vi "1762AdiabaticPassageSequenceALLYB.vi"(0 "Interval":dbl=0.02, 1 "Pump Expose Time (us)":dbl=3.0, 5 "Real Cutoff":i32=15, 7 "runs":dbl, 9 "1762 Freq (MHz)":dbl=98.1, 11 "AP Sweep Width (MHz)":dbl=0.8, 12 "Sweep Duration (us)":dbl=500.0, 13 "Power (-12 Max)":dbl=-12.0) -> (4 "Shelved Fraction":dbl=60.0, 6 "Histogram":waveform(i32)(graph)={"t0"=timestamp(22.5 s since 1904-01-01), "dt"=1.0, "Y"=[1, 1, 1, 1, 0, 6, 2, 2, 3, 4, 7, 6, 5, 10, 5, 12, 9, 9, 11, 8, 6, 6, 14, 4, 7, 2, 1, 3, 3, 3, 1, 0, 1, 0, 3, 0, 0, 0, 0, 0, 0, 0, 0, 0, 0, 0, 0, 0, 0, 0, 0, 0, 0, 0, 0, 0, 0, 0, 0, 0, 0, 0, 0, 0, 0, 0, 0, 0, 0, 0, 0, 0, 0, 0, 0, 0, 0, 0, 0, 0, 0, 0, 1, 0, 0, 0, 0, 1, 0, 0, 1, 0, 2, 0, 1, 2, 0, 2, 0, 4, 5, 0, 0, 2, 3, 2, 3, 8, 4, 7, 6, 3, 7, 5, 6, 9, 6, 8, 4, 10, 4, 4, 7, 7, 6, 8, 11, 7, 12, 6, 13, 6, 7, 12, 11, 11, 2, 4, 5, 6, 7, 5, 5, 4, 5, 4, 3, 2, 4, 6, 3, 2, 3, 1, 0, 4, 2, 1, 2, 1, 2, 1, 2, 2, 1, 1, 1, 1, 0, 0, 1, 1, 1, 0, 0, 2, 0, 0, 2]})   [LabVIEW 2009]
uses:
  <vilib>/Utility/file.llb/Write To Spreadsheet File (DBL).vi
panel:
  out "deshelve attempts":dbl
  out "+/-":dbl=0.4472135954999579
  in  "Restart":bool
  out "Shelving Events":dbl=4.0
  out "Cut-off":i32=50
  out "Background":waveform(i32)(graph)={"t0"=timestamp(64.5 s since 1904-01-01), "dt"=1.0, "Y"=[1, 2, 1, 4, 2, 4, 2, 1, 3, 6, 4, 5, 6, 6, 5, 4, 6, 9, 5, 6, 10, 7, 5, 5, 9, 10, 2, 7, 8, 2, 6, 2, 10, 6, 3, 4, 2, 5, 2, 1, 2, 1, 1, 2, 2, 0, 0, 1, 1, 2]}
  out "+ / -":dbl=10.808259218610711
  out "Background":dbl=86.175
  out "Run Number":dbl=6.0
  out "Path":path=path "c:/data/01-11-2009_14-34-35_0.1000001762AdiabaticPass.txt"
  out "Counts":i32=27
  out "Green":bool=TRUE
  out "Shelved?":bool=TRUE
  out "Red":bool=TRUE
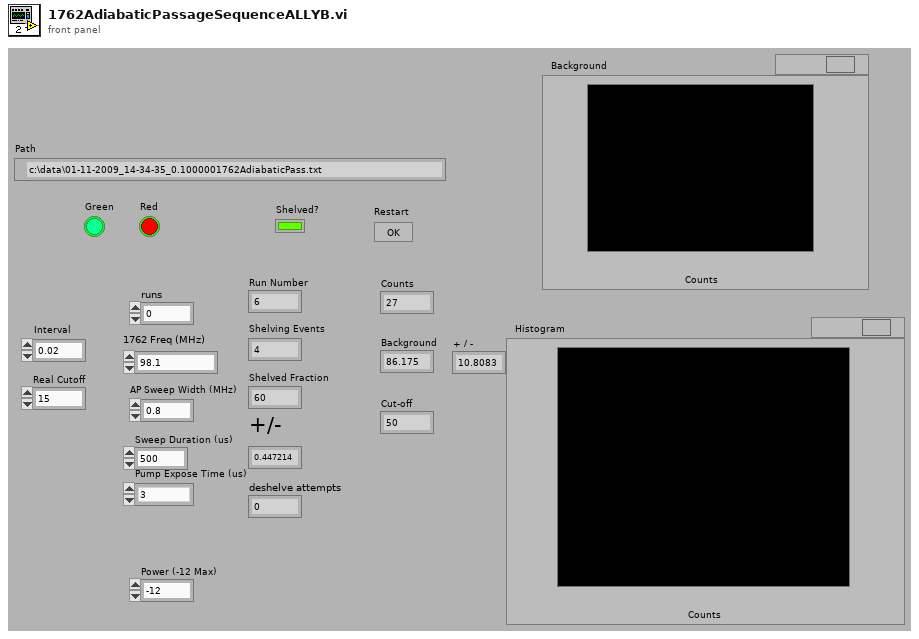
[diagram p1: front panel]
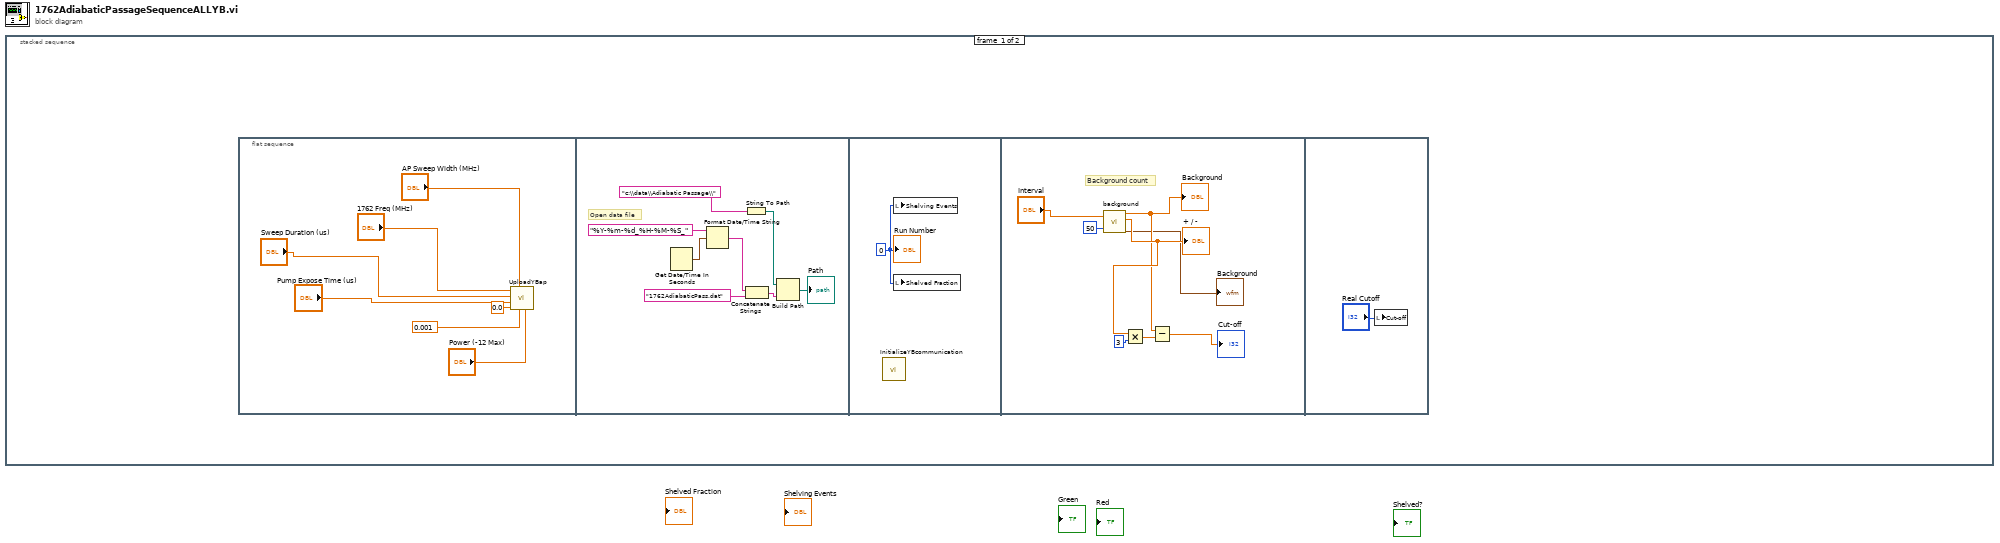
[diagram p0: block diagram]
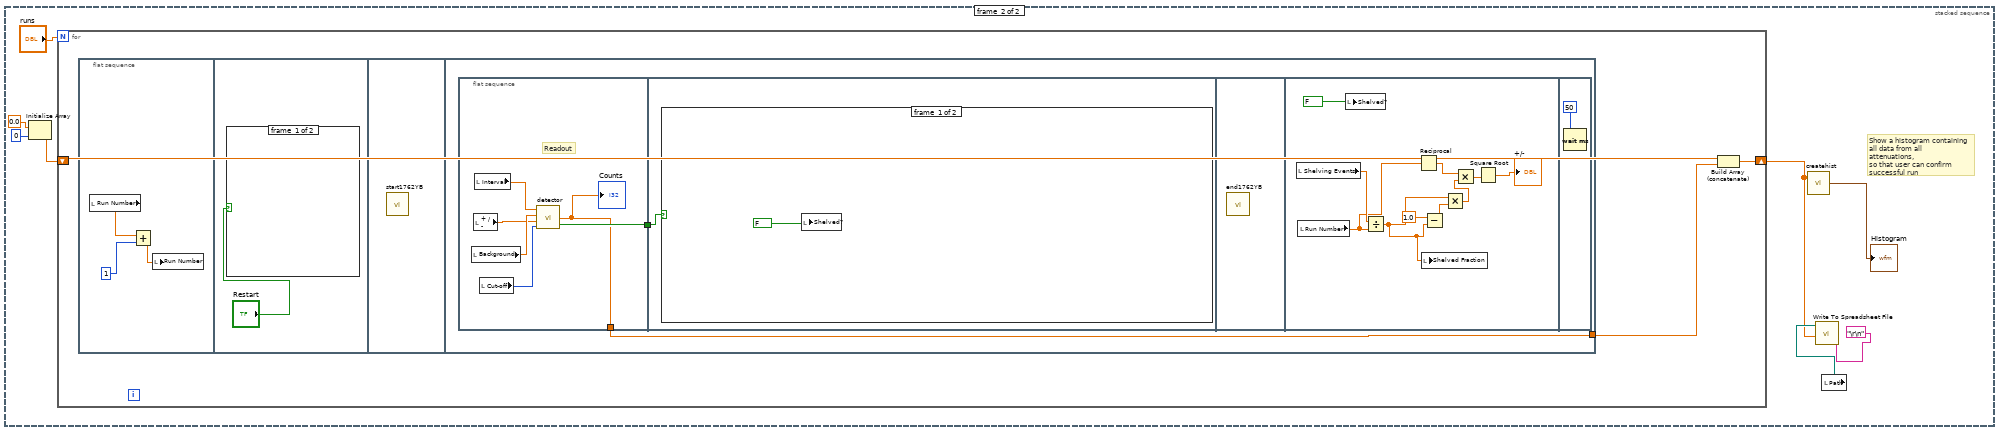
[diagram p2: hidden frame]
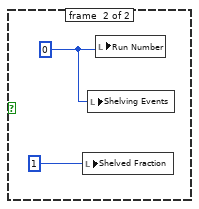
[diagram p3: hidden frame]
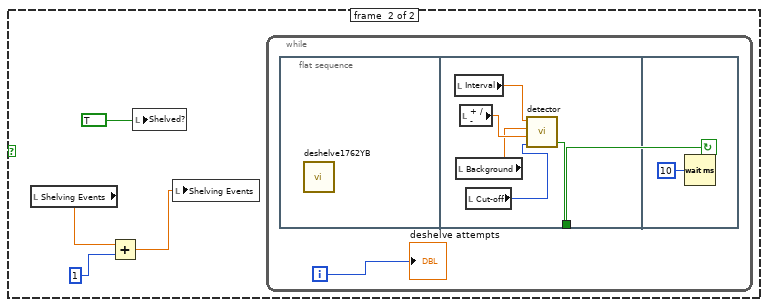
[diagram p4: hidden frame]
diagram:
  n1 = stacked-sequence {
    frame #0 {
      n2 = flat-sequence {
        frame #0 {
          n3 = call "UploadYBap.vi"("Power"="Power (-12 Max)", "AP Freq Step"=0.001, "AP Sweep Width"="AP Sweep Width (MHz)", "1762 RF time"=0.0 ("RF time"), "OP Time"="Pump Expose Time (us)", "1762 Pulse Time"="Sweep Duration (us)", "1762 Frequency"="1762 Freq (MHz)") -> ()  [unwired: 5 in]
        }
        frame #1 {
          # "Open data file"
          n4 = Get Date/Time In Seconds() -> (seconds since 1Jan1904=w13:timestamp)
          n5 = Format Date/Time String(time format string (%c)="%Y-%m-%d_%H-%M-%S_", seconds (now)=w13) -> (date/time string=w15:string)  [unwired: 1 in]
          n6 = String To Path(string="c:\\data\\Adiabatic Passage\\") -> (path=w11:path)
          n7 = Concatenate Strings(w15, "1762AdiabaticPass.dat") -> (w9:string)
          n8 = Build Path(base path=w11, name or relative path=w9) -> (appended path=→"Path":path)
        }
        frame #2 {
          w16 = 0
          n9 = call "InitializeYBcommunication.vi"() -> ()  [unwired: 12 in]
          n10 = local write "Shelving Events"(w16) -> ()
          n11 = local write "Shelved Fraction"(w16) -> ()
          "Run Number" <- w16
        }
        frame #3 {
          # "Background count"
          n12 = call "background.vi"("Interval"="Interval", "Runs"=50) -> ("Mean"=w21:dbl, "Deviation"=w24:dbl, "Histogram"=→"Background":waveform(i32))  [unwired: 1 out]
          "Background" <- w21
          "+ / -" <- w24
          n13 = Multiply(x=w24, y=3) -> (x*y=w22:dbl)
          n14 = Subtract(x=w21, y=w22) -> (x-y=→"Cut-off":dbl)
        }
        frame #4 {
          n15 = local write "Cut-off"("Real Cutoff") -> ()
        }
      }
    }
    frame #1 {
      # "Show a histogram containing\nall data from all attenuations, \nso that user can confirm successful run"
      n16 = Initialize Array(0.0, 0) -> (w29:dbl[])
      n17 = for {
        N: "runs" -> [_]
        shift-right: [w34] -> w27
        shift-left: w29 -> [w35]
        n18 = flat-sequence {
          tunnel: [w43] -> w36
          frame #0 {
            n19 = local read "Run Number"() -> (w37:dbl)
            n20 = Add(x=w37, y=1) -> (x+y=w38:dbl)
            n21 = local write "Run Number"(w38) -> ()
          }
          frame #1 {
            n22 = case shown="True" "Restart" {
              frame #0 {
              }
              frame #1 {
                w42 = 0
                n23 = local write "Shelved Fraction"(1) -> ()
                n24 = local write "Shelving Events"(w42) -> ()
                n25 = local write "Run Number"(w42) -> ()
              }
            }
          }
          frame #2 {
            n26 = call "start1762YB.vi"() -> ()  [unwired: 11 in, 1 out]
          }
          frame #3 {
            n27 = flat-sequence {
              tunnel: [w47] -> w44
              tunnel: [w46] -> w43
              tunnel: w44 -> [w51]
              frame #0 {
                # "Readout"
                n28 = local read "Background"() -> (w50:dbl)
                n29 = local read "+ / -"() -> (w49:dbl)
                n30 = local read "Interval"() -> (w48:dbl)
                n31 = local read "Cut-off"() -> (w45:i32)
                n32 = call "detector.vi"("Cutoff"=w45, "+ / -"=w49, "Background"=w50, "Interval"=w48) -> ("Boolean"=w47:bool, "Counts"=w46:dbl)  [unwired: 1 in]
                "Counts" <- w46
              }
              frame #1 {
                n33 = case shown="True" w51 {
                  frame #0 {
                    n34 = local write "Shelved?"(FALSE) -> ()
                  }
                  frame #1 {
                    n35 = local read "Shelving Events"() -> (w55:dbl)
                    n36 = Add(x=w55, y=1) -> (x+y=w54:dbl)
                    n37 = local write "Shelved?"(TRUE) -> ()
                    n38 = local write "Shelving Events"(w54) -> ()
                    n39 = while {
                      i -> [w57]
                      stop <- w58 continue-if-true
                      n40 = flat-sequence {
                        tunnel: [w63] -> w58
                        frame #0 {
                          n41 = call "deshelve1762YB.vi"() -> ()  [unwired: 11 in, 1 out]
                        }
                        frame #1 {
                          n42 = local read "Interval"() -> (w60:dbl)
                          n43 = local read "Background"() -> (w61:dbl)
                          n44 = local read "+ / -"() -> (w62:dbl)
                          n45 = local read "Cut-off"() -> (w59:i32)
                          n46 = call "detector.vi"("Cutoff"=w59, "+ / -"=w62, "Background"=w61, "Interval"=w60) -> ("Boolean"=w63:bool)  [unwired: 1 in, 1 out]
                        }
                        frame #2 {
                          n47 = Wait (ms)(milliseconds to wait=u32 10) -> ()  [unwired: 1 out]
                        }
                      }
                      "deshelve attempts" <- w57
                    }
                  }
                }
              }
              frame #2 {
                n48 = call "end1762YB.vi"() -> ()  [unwired: 1 in]
              }
              frame #3 {
                n49 = local read "Shelving Events"() -> (w68:dbl)
                n50 = local read "Run Number"() -> (w67:dbl)
                n51 = local write "Shelved?"(FALSE) -> ()
                n52 = Divide(x=w68, y=w67) -> (x/y=w66:dbl)
                n53 = Reciprocal(x=w67) -> (1/x=w73:dbl)
                n54 = local write "Shelved Fraction"(w66) -> ()
                n55 = Subtract(x=1.0, y=w66) -> (x-y=w71:dbl)
                n56 = Multiply(x=w66, y=w71) -> (x*y=w69:dbl)
                n57 = Multiply(x=w73, y=w69) -> (x*y=w72:dbl)
                n58 = Square Root(x=w72) -> (sqrt(x)=→"+/-":dbl)
              }
              frame #4 {
                n59 = Wait (ms)(milliseconds to wait=u32 50) -> ()  [unwired: 1 out]
              }
            }
          }
        }
        n60 = Build Array (concatenate)(w35, w36) -> (w34:dbl[])
      }
      n61 = call "createhist.vi"("Array"=w27) -> ("Waveform Graph"=→"Histogram":waveform(i32))  [unwired: 1 in]
      n62 = local read "Path"() -> (w33:path)
      n63 = call-poly <vilib>:"Write To Spreadsheet File.vi"("delimiter (\\t)"="\r\n", "1D data"=w27, "file path (dialog if empty)"=w33) -> ()  [unwired: 5 in, 1 out]
    }
  }
